vi "getSettingControlReferences.vi"(11 "Setting in":refnum<class "Setting.lvclass">) -> (2 "SettingControlReferences":refnum<vi>[](array[refnum]), 3 "Setting out":refnum<class "Setting.lvclass">)   [LabVIEW 2016, in "Settings.lvlib" / "Setting.lvclass"]
uses:
  Setting.lvclass
  Setting.lvclass/Setting.ctl
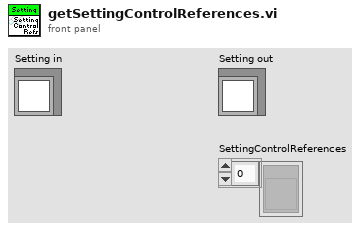
[diagram p1: front panel]
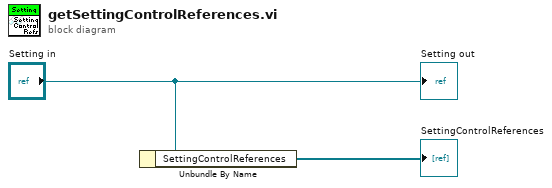
[diagram p0: block diagram]
diagram:
  n1 = Unbundle By Name("Setting in") -> ("SettingControlReferences"=→"SettingControlReferences":refnum<vi>[])
  "Setting out" <- "Setting in"
